vi "Cluster_test2.vi"() -> ()   [LabVIEW 2018]
panel:
  out "배열":dbl[](array[numeric])
  in  "추가된 배열 2":dbl[](array[numeric])
  out "추가된 배열":dbl[](array[numeric])
  in  "숫자형 4":dbl
  in  "숫자형 3":dbl
  in  "숫자형 2":dbl
  in  "숫자형":dbl
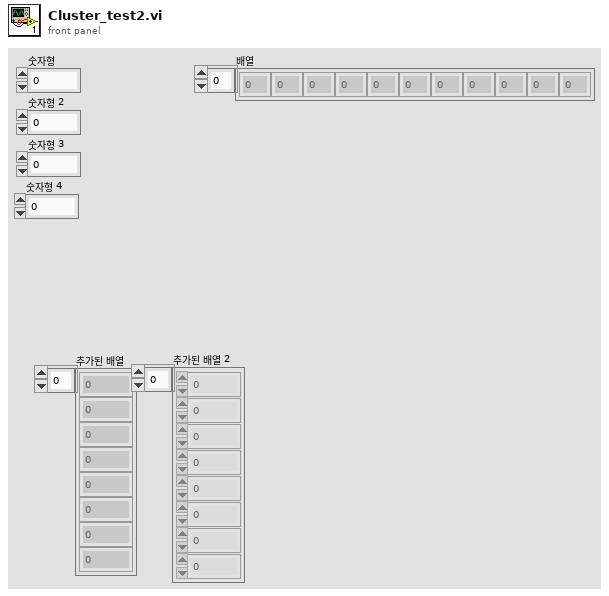
[diagram p1: front panel]
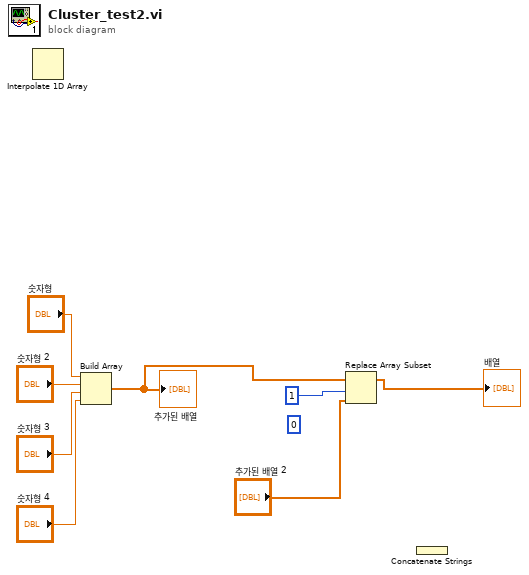
[diagram p0: block diagram]
diagram:
  (unwired) 0 ("인덱스")
  n1 = Interpolate 1D Array() -> ()  [unwired: 2 in, 1 out]
  n2 = Build Array("숫자형", "숫자형 2", "숫자형 3", "숫자형 4") -> (w4:dbl[])
  "추가된 배열" <- w4
  n3 = Replace Array Subset(array=w4, new element="추가된 배열 2", index=1 ("인덱스")) -> (→"배열":dbl[])
  n4 = Concatenate Strings() -> ()  [unwired: 1 in, 1 out]
